vi "RichToFlatgoogle_protobuf_SourceContext.vi"(5 "OutputClusterType":T1, 11 "InputCluster":T2) -> (3 "OutputCluster":T1)   [LabVIEW 2021, in "ni.measurementlink.measurement.v1.api.lvlib"]
uses:
  ni.measurementlink.measurement.v1.api.lvlib
  google_protobuf_SourceContext.ctl
  google_protobuf_SourceContext_Flat.ctl
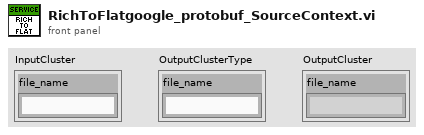
[diagram p1: front panel]
types:
  T1 = typedef "ni.measurementlink.measurement.v1.api.lvlib/google_protobuf_SourceContext_Flat.ctl" = cluster{"file_name":string}
  T2 = typedef "ni.measurementlink.measurement.v1.api.lvlib/google_protobuf_SourceContext.ctl" = cluster{"file_name":string}
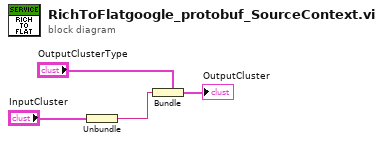
[diagram p0: block diagram]
diagram:
  n1 = Unbundle "Unbundle"("InputCluster") -> ("file_name"=w1:string)
  n2 = Bundle "Bundle"(cluster="OutputClusterType", "file_name"=w1) -> (→"OutputCluster":T1)
